vi "SP Calculate Scaling Factors.vi"(9 "X-Y Plot":cluster{"X":dbl[], "Y":dbl[]}[](array[cluster]), 10 "CH Control":T1={"Trace On"=TRUE, "Measure"=0, "Format"=0, "Autoscale"=TRUE, "Reference"=0.0, "\nRefUnit"="dB/Div", "Position"=5.0, "Scale"=10.0, "ScaleUnit"="dB/Div", "LimitOn"=TRUE, "LimitFill"=FALSE, "Display Data"=0, "Show Markers"=TRUE, "SXX"=""} {"Reference" format="%#.2g"; "Display Data" items=["Data", "Memory", "Data/Memory"]; "Format" items=["Log Mag", "Phase", "Expanded Phase", "Delay", "Smith", "Polar", "Lin Mag", "SWR", "Loss", "Real", "Imaginary"]; "Scale" min=0.001 step=1.0 format="%#.2g"; "Position" min=0.0 max=10.0}, 11 "Autoscale?":bool) -> (0 "Y Min":dbl, 1 "Y Max":dbl, 2 "Scale":dbl, 3 "Reference":dbl, 4 "Y Markers":dbl[](array[numeric]))   [LabVIEW 2011]
uses:
  TypeDefs/SP Display Trace Controls.ctl
  TypeDefs/SP Display Format.ctl
  TypeDefs/SP Display Data.ctl
panel:
  # "Div"
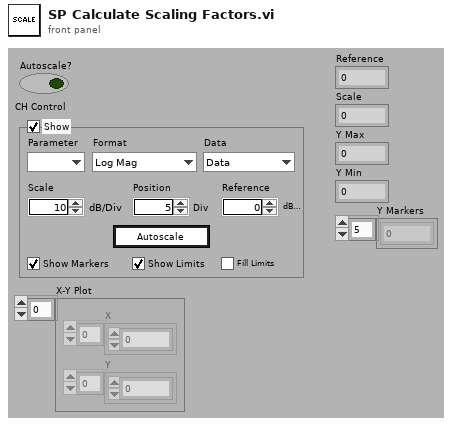
[diagram p1: front panel]
types:
  T1 = typedef "SP Display Trace Controls.ctl" = cluster{"Trace On":bool, "Measure":i32, "Format":T2, "Autoscale":bool, "Reference":dbl, "\nRefUnit":string, "Position":dbl, "Scale":dbl, "ScaleUnit":string, "LimitOn":bool, "LimitFill":bool, "Display Data":T3, "Show Markers":bool, "SXX":string}
  T2 = typedef "SP Display Format.ctl" = i32
  T3 = typedef "SP Display Data.ctl" = u16
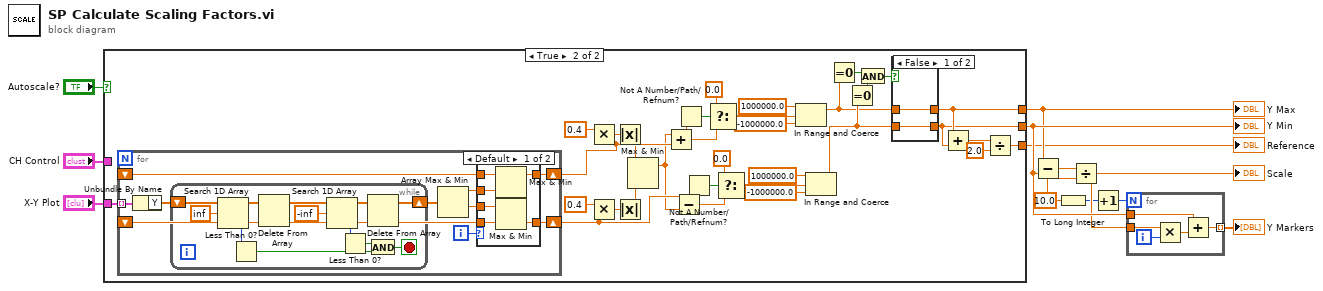
[diagram p0: block diagram]
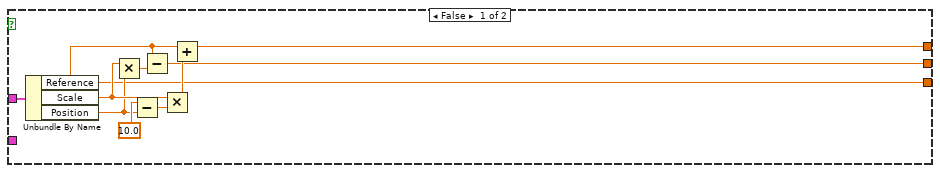
[diagram p2: hidden frame]
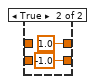
[diagram p4: hidden frame]
diagram:
  w6 = 10.0
  n1 = case shown="True" "Autoscale?" {
    tunnel: [w15 w25] -> w8
    tunnel: [w14 w24] -> w9
    tunnel: "X-Y Plot" -> [_ w31]
    tunnel: "CH Control" -> [w22 _]
    tunnel: [w13 w27] -> w1
    frame False {
      n2 = Unbundle By Name(w22) -> ("Reference"=w13:dbl, "Scale"=w17:dbl, "Position"=w16:dbl)
      n3 = Multiply(x=w17, y=w16) -> (x*y=w19:dbl)
      n4 = Subtract(x=10.0, y=w16) -> (x-y=w21:dbl)
      n5 = Subtract(x=w13, y=w19) -> (x-y=w14:dbl)
      n6 = Multiply(x=w17, y=w21) -> (x*y=w20:dbl)
      n7 = Add(x=w13, y=w20) -> (x+y=w15:dbl)
    }
    frame True {
      n8 = for {
        tunnel: w31 -> [w64] mode=indexing
        shift-right: [w61] -> w32
        shift-left: _ -> [w59]
        shift-right: [w60] -> w33
        shift-left: _ -> [w58]
        i -> [w57]
        n9 = Unbundle By Name(w64) -> ("Y"=w56:dbl[])
        n10 = while {
          shift-right: [w65] -> w55
          shift-left: w56 -> [w73]
          stop <- w66 stop-if-true
          n11 = Search 1D Array(1D array=w73, element=inf) -> (index of element=w70:i32)  [unwired: 1 out]
          n12 = Less Than 0?(x=w70) -> (x < 0?=w67:bool)
          n13 = Delete From Array(array=w73, index=w70) -> (array with subset deleted=w71:dbl[])  [unwired: 1 in, 1 out]
          n14 = Search 1D Array(1D array=w71, element=-inf) -> (index of element=w69:i32)  [unwired: 1 out]
          n15 = Less Than 0?(x=w69) -> (x < 0?=w68:bool)
          n16 = Delete From Array(array=w71, index=w69) -> (array with subset deleted=w65:dbl[])  [unwired: 1 in, 1 out]
          n17 = And(x=w68, y=w67) -> (x .and. y?=w66:bool)
        }
        n18 = Array Max & Min(array=w55) -> (max value=w63:dbl, min value=w62:dbl)  [unwired: 2 out]
        n19 = case shown="Default" w57 {
          tunnel: w63 -> [w75 w82]
          tunnel: w62 -> [w79 w81]
          tunnel: [w80 w82] -> w61
          tunnel: [w78 w81] -> w60
          tunnel: w59 -> [w76 _]
          tunnel: w58 -> [w77 _]
          frame Default {
            n20 = Max & Min(x=w76, y=w75) -> (max(x,y)=w80:dbl)  [unwired: 1 out]
            n21 = Max & Min(x=w79, y=w77) -> (min(x,y)=w78:dbl)  [unwired: 1 out]
          }
          frame 0 {
          }
        }
      }
      n22 = Multiply(x=0.4, y=w32) -> (x*y=w52:dbl)
      n23 = Multiply(x=0.4, y=w33) -> (x*y=w51:dbl)
      n24 = Absolute Value(x=w52) -> (abs(x)=w30:dbl)
      n25 = Absolute Value(x=w51) -> (abs(x)=w29:dbl)
      n26 = Max & Min(x=w30, y=w29) -> (max(x,y)=w28:dbl)  [unwired: 1 out]
      n27 = Add(x=w28, y=w32) -> (x+y=w42:dbl)
      n28 = Subtract(x=w33, y=w28) -> (x-y=w43:dbl)
      n29 = Not A Number/Path/Refnum?(number/path/refnum=w42) -> (NaN/Path/Refnum?=w47:bool)
      n30 = Not A Number/Path/Refnum?(number/path/refnum=w43) -> (NaN/Path/Refnum?=w44:bool)
      n31 = Select(t=0.0, s=w47, f=w42) -> (s? t:f=w35:dbl)
      n32 = Select(t=0.0, s=w44, f=w43) -> (s? t:f=w39:dbl)
      n33 = In Range and Coerce(upper limit=1000000.0, x=w35, lower limit=-1000000.0) -> (coerced(x)=w34:dbl)  [unwired: 1 out]
      n34 = In Range and Coerce(upper limit=1000000.0, x=w39, lower limit=-1000000.0) -> (coerced(x)=w38:dbl)  [unwired: 1 out]
      n35 = Equal To 0?(x=w34) -> (x = 0?=w49:bool)
      n36 = Equal To 0?(x=w38) -> (x = 0?=w50:bool)
      n37 = And(x=w49, y=w50) -> (x .and. y?=w48:bool)
      n38 = case shown="False" w48 {
        tunnel: w38 -> [w83 _]
        tunnel: w34 -> [w84 _]
        tunnel: [w84 1.0] -> w25
        tunnel: [w83 -1.0] -> w24
        frame False {
        }
        frame True {
        }
      }
      n39 = Add(x=w25, y=w24) -> (x+y=w23:dbl)
      n40 = Divide(x=w23, y=2.0) -> (x/y=w27:dbl)
    }
  }
  "Y Min" <- w9
  "Y Max" <- w8
  "Reference" <- w1
  n41 = Subtract(x=w8, y=w9) -> (x-y=w5:dbl)
  n42 = To Long Integer(number=w6) -> (32bit integer=w4:i32)
  n43 = Divide(x=w5, y=w6) -> (x/y=w7:dbl)
  "Scale" <- w7
  n44 = Increment(x=w4) -> (x+1=w2:i32)
  n45 = for {
    N: w2 -> [_]
    tunnel: w9 -> [w90]
    tunnel: w7 -> [w91]
    tunnel: [w88] -> w3 mode=indexing
    i -> [w87]
    n46 = Multiply(x=w91, y=w87) -> (x*y=w89:dbl)
    n47 = Add(x=w90, y=w89) -> (x+y=w88:dbl)
  }
  "Y Markers" <- w3
